vi "exercice6-1.vi"() -> ()   [LabVIEW 2013]
panel:
  out "Racine":dbl
  in  "Valeur":dbl
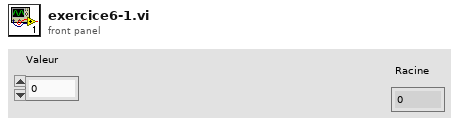
[diagram p1: front panel]
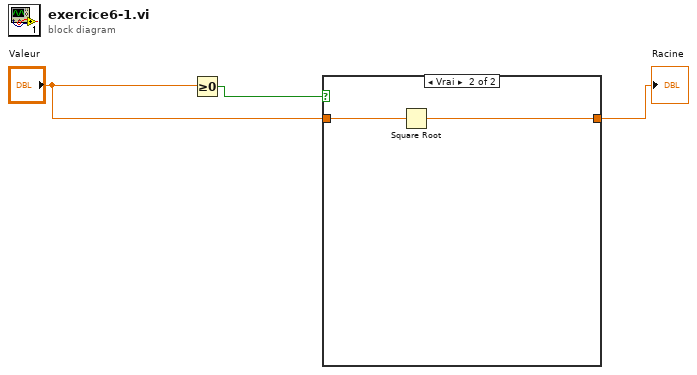
[diagram p0: block diagram]
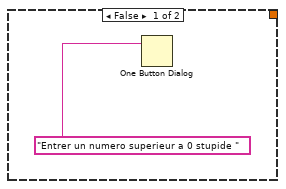
[diagram p2: hidden frame]
diagram:
  n1 = Greater Or Equal To 0?(x="Valeur") -> (x >= 0?=w3:bool)
  n2 = case shown="Vrai" w3 {
    tunnel: "Valeur" -> [_ w6]
    tunnel: [_ w5] -> w1
    frame False {
      n3 = One Button Dialog(message="Entrer un numero superieur a 0 stupide ") -> ()  [unwired: 1 in, 1 out]
    }
    frame True {
      n4 = Square Root(x=w6) -> (sqrt(x)=w5:dbl)
    }
  }
  "Racine" <- w1
